vi "PCO_ConvertSetBayer.vi"(8 "error in (no error)":errorcluster {"code" format="%x"}, 10 "strBayer":cluster{"iKernel":i32, "iColorMode":i32} {"iKernel" items=["BAYER_UPPER_LEFT_IS_RED", "BAYER_UPPER_LEFT_IS_GREEN_RED", "BAYER_UPPER_LEFT_IS_GREEN_BLUE", "BAYER_UPPER_LEFT_IS_BLUE"]}, 11 "ph":u64) -> (0 "error out":errorcluster {"code" format="%x"}, 2 "ErrorMessage":i32 format="%x", 3 "ph out":u64)   [LabVIEW 2019, in "Convert.lvlib"]
doc: "int PCOCONVERT_API PCO_ConvertSetBayer(HANDLE ph, PCO_Bayer* pstrBayer);"
uses:
  Convert.lvlib
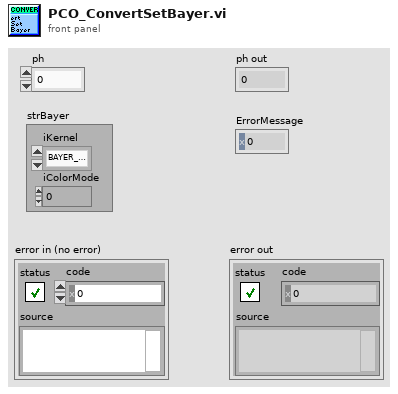
[diagram p1: front panel]
types:
  T1 = cluster{"wSize":u16, "wDummy":u16, "iKernel":i32, "iColorMode":i32, "dwzzDummy1":cluster{u32, u32, u32, u32, u32, u32, u32, u32, u32, u32, u32, u32, u32, u32, u32, u32, u32, u32, u32, u32, u32, u32, u32, u32, u32, u32, u32, u32, u32, u32, u32, u32, u32, u32, u32, u32, u32, u32, u32, u32, u32, u32, u32, u32, u32, u32, u32, u32, u32, u32, u32, u32, u32, u32, u32, u32, u32, u32, u32, u32, u32}}
  T2 = cluster{u32, u32, u32, u32, u32, u32, u32, u32, u32, u32, u32, u32, u32, u32, u32, u32, u32, u32, u32, u32, u32, u32, u32, u32, u32, u32, u32, u32, u32, u32, u32, u32, u32, u32, u32, u32, u32, u32, u32, u32, u32, u32, u32, u32, u32, u32, u32, u32, u32, u32, u32, u32, u32, u32, u32, u32, u32, u32, u32, u32, u32}
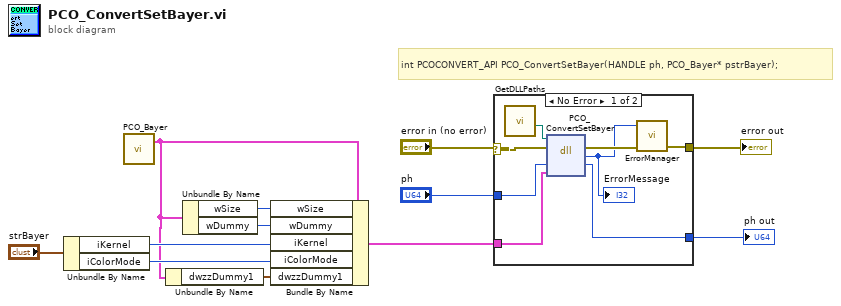
[diagram p0: block diagram]
diagram:
  # "int PCOCONVERT_API PCO_ConvertSetBayer(HANDLE ph, PCO_Bayer* pstrBayer);"
  n1 = Unbundle By Name("strBayer") -> ("iKernel"=w7:i32, "iColorMode"=w6:i32)
  n2 = call "PCO_Bayer.vi"() -> ("PCO_Bayer_Raw"=w3:T1)  [unwired: 4 in, 3 out]
  n3 = Unbundle By Name(w3) -> ("dwzzDummy1"=w2:T2)
  n4 = Unbundle By Name(w3) -> ("wSize"=w5:u16, "wDummy"=w4:u16)
  n5 = Bundle By Name(cluster=w3, "wSize"=w5, "wDummy"=w4, "iKernel"=w7, "iColorMode"=w6, "dwzzDummy1"=w2) -> (w1:T1)
  n6 = case shown="No Error" "error in (no error)" {
    selector: "error in (no error)" -> [w17 w22]
    tunnel: "ph" -> [w20 w21]
    tunnel: [w19 w21] -> w11
    tunnel: w1 -> [w18 _]
    tunnel: [w15 w22] -> w10
    frame No Error {
      n7 = call "GetDLLPaths.vi"() -> ("PCO_Conv_Path"=w13:path)  [unwired: 9 in, 2 out]
      n8 = dll-call lib="?" fn="PCO_ConvertSetBayer"(path in=w13, error in=w17, "ph"=w20, "pstrBayer"=w18) -> (error out=w16:errorcluster, "return type"=w14:i32, "ph"=w19:u64)  [unwired: 2 in, 1 out]
      "ErrorMessage" <- w14
      n9 = call "ErrorManager.vi"("error in (no error)"=w16, "error code"=w14) -> ("error out"=w15:errorcluster)  [unwired: 3 in]
    }
    frame Error {
    }
  }
  "ph out" <- w11
  "error out" <- w10
